vi "heating_visu.vi"(7 "name":string="HT1", 9 "stop":bool, 10 "connect (T)":bool=TRUE, 11 "ZY_In":T4={"Z"={"Z_Source"=enum."local disabled", "Z_SetState"=enum."on", "Z_State"=enum."alarm", "Z_State_T"=0, "ZM_State"=enum."initialization", "ZM_State_T"=0, "ALR  L1"=FALSE, "ALR  L2"=FALSE, "HH_run"=0}, "Y"={"Y_Source"=enum."local disabled", "Y_SetState"=enum."auto", "SP_Set"=0.0, "SP"=0.0, "PV"=0.0, "Y_Set"=0.0, "Y"=0.0, "Y_State"={"code"=0, "visible"=FALSE, "color"=0}, "YB"=FALSE}, "ALR_Status"=[]} {"Y"."Y_Set" format="%.2f"; "Y"."SP" step=0.01 format="%.2f"; "Y"."Y" format="%.2f"; "Y"."PV" step=0.01 format="%.2f"; "Y"."SP_Set" step=0.01 format="%.2f"}) -> (2 "Write Enable":bool, 3 "ZY_out":T1={"Z_HSw"=1, "Z_HSetState"=enum."on", "Y_HSw"=1, "Y_HSetState"=enum."auto", "SP"=0.0, "Y_H"=0.0, "Reset_ALR"=FALSE} {"Y_H" step=1.0; "SP" step=0.01 format="%.2f"}, 5 "This VI":refnum<vi>)   [LabVIEW 2019, in "Heating.lvlib"]
uses:
  Heating.lvlib
  Inputs/Ctl/Parameter State.ctl
  ctl/ZY_state_short.ctl
  ctl/Z.ctl
  ctl/Z_source.ctl
  ctl/Z_State.ctl
  ctl/ZM_State.ctl
  ctl/Y_short.ctl
  ctl/Y_source.ctl
  ctl/Y_state.ctl
  Inputs/Ctl/Parameter State short.ctl
  Alarms/Ctl/ALR_Status_short.ctl
  ctl/ZY_control.ctl
  Logik/fronts.vi
  Trigers/RS.vi
  Trigers/D^.vi
  Timer Delay/Timer.vi
  Counter/Generator simplified.vi
  Global stop.vi
  Change_state.vi
  Timer Delay/Timers.lvlib
  Counter/Counter.lvlib
  Inputs/Inputs.lvlib
  Alarms/Alarms.lvlib
panel:
  in  "on_change":bool
  in  "SP_change":bool
  in  "Y_change":bool
  in  "Z_HSwitch":bool
  out "Z1 ind":u8(ring)
  in  "PV_State":T12
  out "T stage":dbl format="%<%M:%S>t"
  in  "manual control":dbl(slide)=25.0 caption="%" min=0.0 max=100.0 step=1.0 scale=0.0..100.0 scale format="%#.1f"
  out "Z3 ind":u16(ring)
  in  "setpoint":cluster{dbl, dbl}(slide)={350.0, 0.0} caption="oC" scale=0.0..500.0 scale format="%#.1f"
  out "PV":dbl(slide) caption="oC" scale=0.0..500.0 scale format="%#.1f"
  in  "on":bool=TRUE
  in  "ALRL1_reset":bool
  in  "ALRL2_reset":bool
  in  "Y_HSwitch":bool=TRUE
  out "Y ind":u8(ring)
  out "Z5 State":string
  out "Y output":dbl format="%.2f"
  # "PV"
  # "SP"
  # "Y"
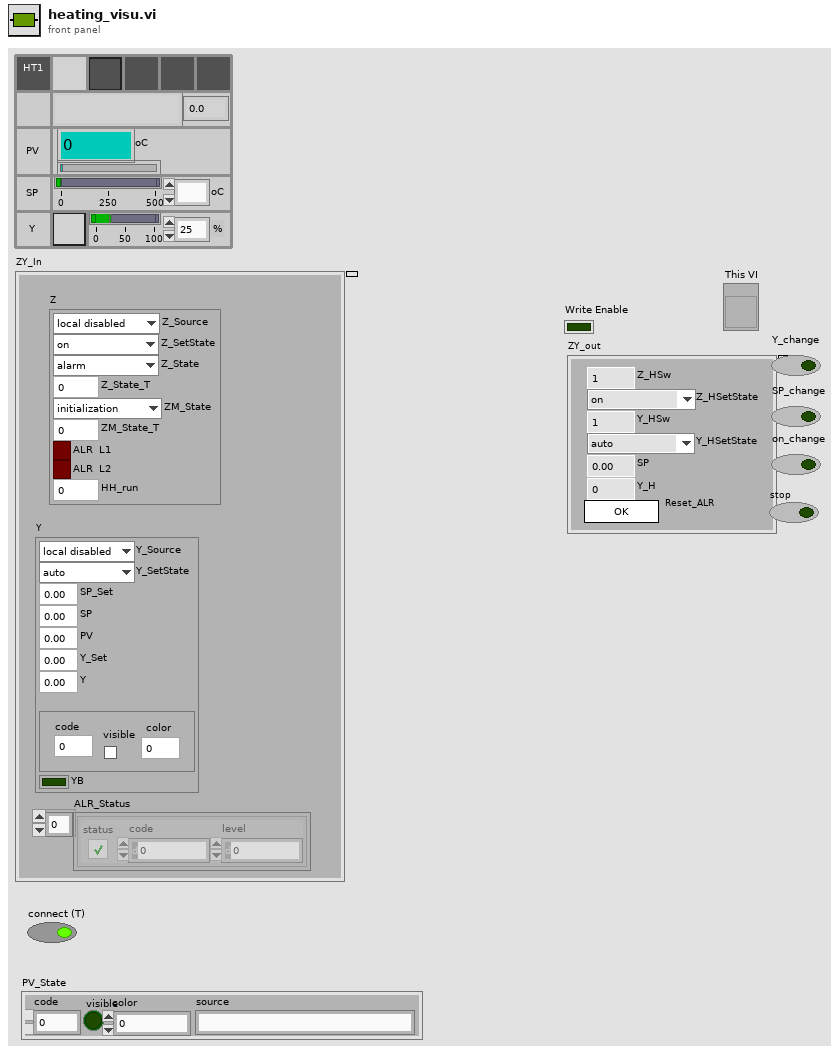
[diagram p1: front panel]
types:
  T1 = typedef "Heating.lvlib/ZY_control.ctl" = cluster{"Z_HSw":u8, "Z_HSetState":T2, "Y_HSw":u8, "Y_HSetState":T3, "SP":dbl, "Y_H":dbl, "Reset_ALR":bool}
  T2 = typedef "Heating.lvlib/Z_State.ctl" = enum8{"initialization", "alarm", "disabled", "not ready", "stop ready", "reserv", "switched off", "reserv2", "switched on", "check", "on min", "decrease out", "on", "increase out", "on max"}
  T3 = typedef "Heating.lvlib/Y_state.ctl" = enum8{"initialize", "alarm", "min", "stop", "hand", "auto", "max"}
  T4 = typedef "Heating.lvlib/ZY_state_short.ctl" = cluster{"Z":T5, "Y":T8, "ALR_Status":T11[]}
  T5 = typedef "Heating.lvlib/Z.ctl" = cluster{"Z_Source":T6, "Z_SetState":T2, "Z_State":T2, "Z_State_T":u32, "ZM_State":T7, "ZM_State_T":u32, "ALR  L1":bool, "ALR  L2":bool, "HH_run":u64}
  T6 = typedef "Heating.lvlib/Z_source.ctl" = enum8{"initialize", "local disabled", "local hand", "hand", "auto", "dist"}
  T7 = typedef "Heating.lvlib/ZM_State.ctl" = enum8{"initialization", "stop", "start_cmd", "contactor_on_cmd", "heating", "on", "stop_cmd", "power_down", "contactor_off_cmd", "cooling", "restart_delay"}
  T8 = typedef "Heating.lvlib/Y_short.ctl" = cluster{"Y_Source":T9, "Y_SetState":T3, "SP_Set":dbl, "SP":dbl, "PV":dbl, "Y_Set":dbl, "Y":dbl, "Y_State":T10, "YB":bool}
  T9 = typedef "Heating.lvlib/Y_source.ctl" = enum8{"initialize", "local disabled", "local hand", "hand", "auto", "dist"}
  T10 = typedef "Inputs.lvlib/Parameter State short.ctl" = cluster{"code":i32, "visible":bool, "color":u32}
  T11 = typedef "Alarms.lvlib/ALR_Status_short.ctl" = cluster{"status":bool, "code":i32, "level":i32}
  T12 = typedef "Inputs.lvlib/Parameter State.ctl" = cluster{"code":i32, "visible":bool, "color":u32, "source":string}
  T13 = enum32{"Invalid Status", "Unconnected", "Active", "Idle", "Error", "Connecting"}
  T14 = enum8{"Enabled", "Disabled", "Disabled and Grayed Out"}
  T15 = typedef "LVDataSocketStatusTypeDef.ctl" = cluster{"Code":enum32{"Invalid Status", "Unconnected", "Active", "Idle", "Error", "Connecting"}, "Text":string}
  T16 = cluster{"Write":bool, "Z1_ind":u8, "Z1_ind_blinking":bool, "Z_HSwitch_out":bool, "Z_HSwitch_visible":bool, "Z_HSwitch_disabled":enum8{"Enabled", "Disabled", "Disabled and Grayed Out"}}
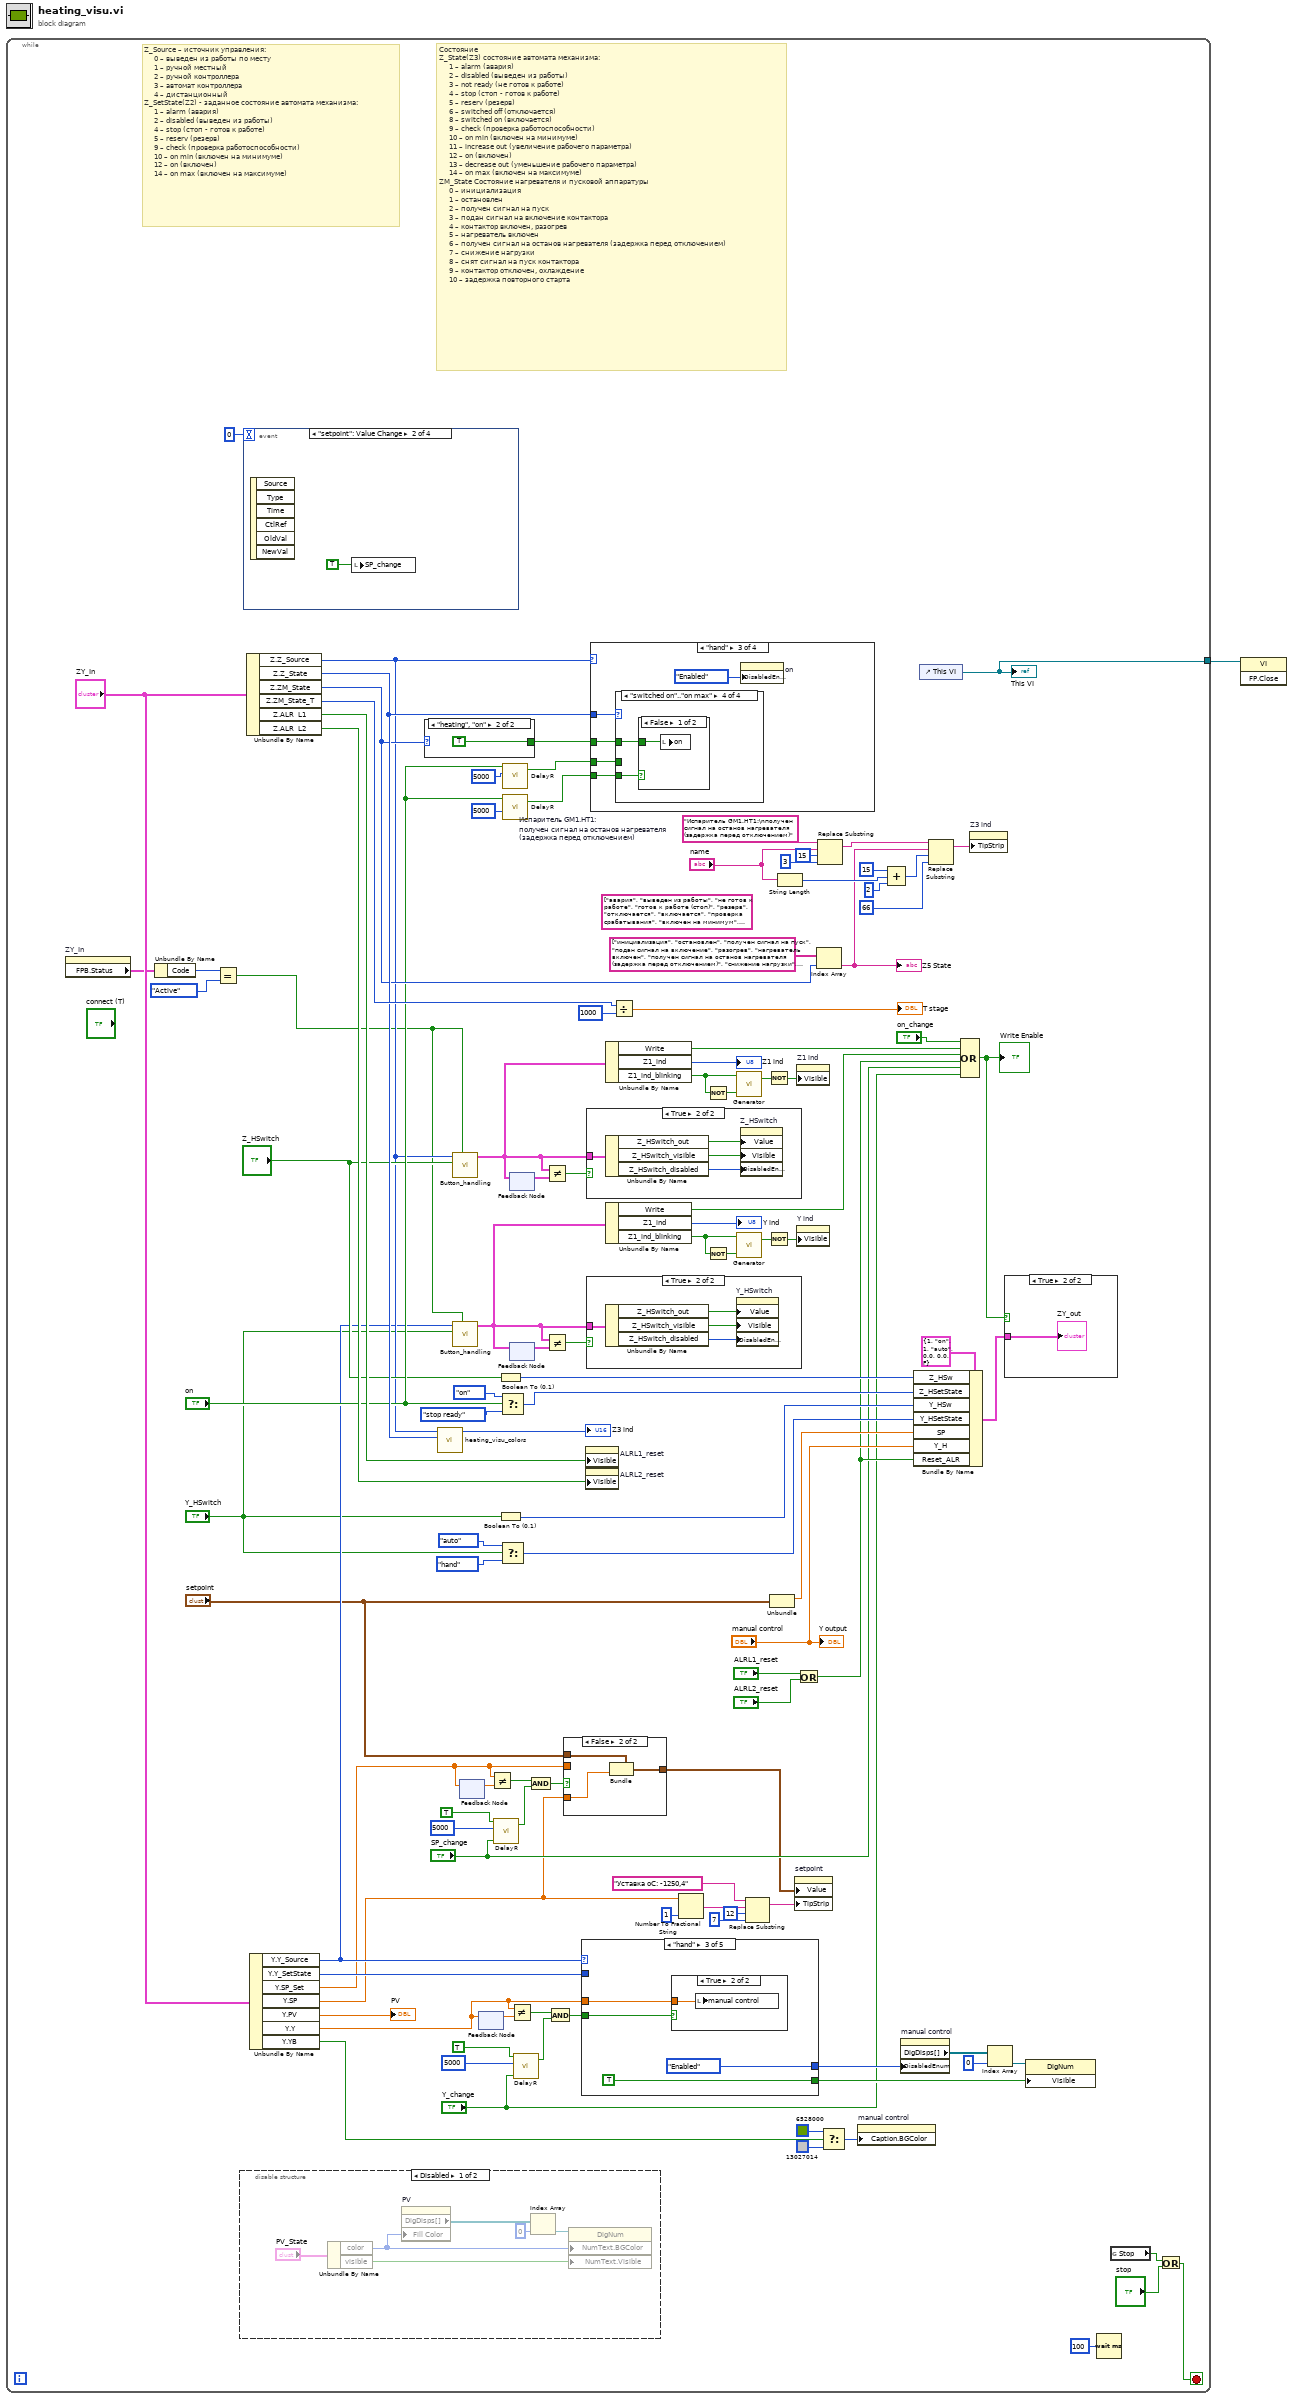
[diagram p0: block diagram]
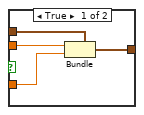
[diagram p3: hidden frame]
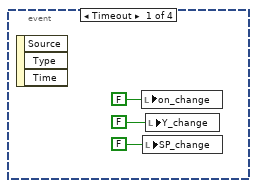
[diagram p4: hidden frame]
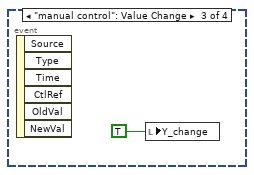
[diagram p5: hidden frame]
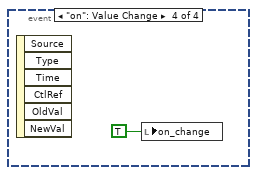
[diagram p6: hidden frame]
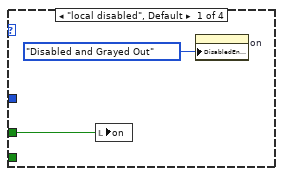
[diagram p8: hidden frame]
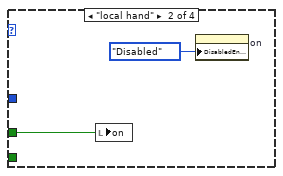
[diagram p9: hidden frame]
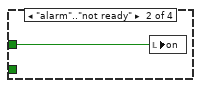
[diagram p11: hidden frame]
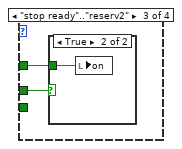
[diagram p12: hidden frame]
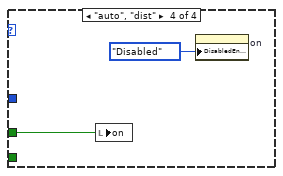
[diagram p15: hidden frame]
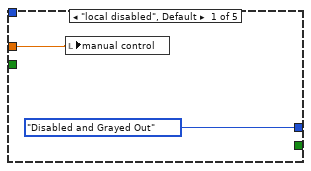
[diagram p19: hidden frame]
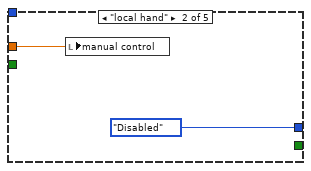
[diagram p20: hidden frame]
diagram:
  n1 = while {
    tunnel: [w2] -> w1
    stop <- w9 stop-if-true
    (unwired) string[] ["авария", "выведен из работы", "не готов к работе", "готов к работе (стоп)", "резерв", "отключается", "включается", "проверка срабатывания", "включен на минимум", "увеличение произв", "включен", "уменьшение произв", "включен на максимум"]
    w106 = "Испаритель GM1.HT1:\nполучен сигнал на останов нагревателя (задержка перед отключением)"  # Испаритель GM1.HT1: получен сигнал на останов нагревателя (задержка перед отключением)
    # "Z_Source – источник управления:\n     0 – выведен из работы по месту\n     1 – ручной местный\n     2 – ручной контроллера\n     3 – автомат контроллера\n     4 – дистанционный\nZ_SetState(Z2) - заданное состояние автомата механизма:\n     1 – alarm (авария)\n     2 – disabled (выведен из работы)\n     4 – stop (стоп - готов к работе)\n     5 – reserv (резерв)\n     9 – check (проверка работоспособности)\n     10 – on min (включен на минимуме)\n     12 – on (включен)\n     14 – on max (включен на максимуме)"
    # "Состояние\nZ_State(Z3) состояние автомата механизма:\n     1 – alarm (авария)\n     2 – disabled (выведен из работы)\n     3 – not ready (не готов к работе)\n     4 – stop (стоп - готов к работе)\n     5 – reserv (резерв)\n     6 – switched off (отключается)\n     8 – switched on (включается)\n     9 – check (проверка работоспособности)\n     10 – on min (включен на минимуме)\n     11 – increase out (увеличение рабочего параметра)\n     12 – on (включен)\n     13 – decrease out (уменьшение рабочего параметра)\n     14 – on max (включен на максимуме)\nZM_State Состояние нагревателя и пусковой аппаратуры\n     0 – инициализация\n     1 – остановлен\n     2 – получен сигнал на пуск\n     3 – подан сигнал на включение контактора\n     4 – контактор включен, разогрев\n     5 – нагреватель включен\n     6 – получен сигнал на останов нагревателя (задержка перед отключением)\n     7 – снижение нагрузки\n     8 – снят сигнал на пуск контактора\n     9 – контактор отключен, охлаждение\n     10 – задержка повторного старта"
    n2 = property on="ZY_In" class="Clust (strict)"() -> ("FPB.Status"=w6:T15)  [unwired: 2 in, 2 out]
    n3 = Unbundle By Name(w6) -> ("Code"=w5:T13)
    n4 = Equal?(x=w5, y=T13."Active" ("Code")) -> (x = y?=w3:bool)
    n5 = disable-structure shown="Disabled" {
      frame Disabled {
        n6 = Unbundle By Name("PV_State") -> ("color"=w156:u32, "visible"=w157:bool)
        n7 = property on="PV" class="Slide (strict)"("Fill Color"=w156) -> ("DigDisps[]"=w160:refnum<vi>[])  [unwired: 2 in, 2 out]
        n8 = Index Array(array=w160, index=0) -> (element=w158:refnum<vi>)
        n9 = property on="Property Node" class="DigNum"(reference=w158, "NumText.BGColor"=w156, "NumText.Visible"=w157) -> ()  [unwired: 1 in, 2 out]
      }
      frame Enabled {
      }
    }
    n10 = event shown="[1] \"setpoint\": Value Change" {
      selector: _ -> [_ _ _ _]
      dyn-events: _ -> [_ _ _ _]
      timeout: 0 -> [_ _ _ _]
      event Timeout {
        n11 = event-data() -> ()  [unwired: 1 in, 3 out]
        n12 = local write "on_change"(FALSE ("manual_reset")) -> ()
        n13 = local write "SP_change"(FALSE ("manual_reset")) -> ()
        n14 = local write "Y_change"(FALSE ("manual_reset")) -> ()
      }
      event "setpoint": Value Change {
        n15 = event-data() -> ()  [unwired: 1 in, 6 out]
        n16 = local write "SP_change"(TRUE ("manual_reset")) -> ()
      }
      event "manual control": Value Change {
        n17 = event-data() -> ()  [unwired: 1 in, 6 out]
        n18 = local write "Y_change"(TRUE ("manual_reset")) -> ()
      }
      event "on": Value Change {
        n19 = event-data() -> ()  [unwired: 1 in, 6 out]
        n20 = local write "on_change"(TRUE ("manual_reset")) -> ()
      }
    }
    n21 = Unbundle By Name("ZY_In") -> ("Z.Z_Source"=w59:T6, "Z.Z_State"=w78:T2, "Z.ZM_State"=w69:T7, "Z.ZM_State_T"=w83:u32, "Z.ALR  L1"=w82:bool, "Z.ALR  L2"=w81:bool)
    n22 = Unbundle By Name("ZY_In") -> ("Y.Y_Source"=w58:T9, "Y.Y_SetState"=w80:T3, "Y.SP_Set"=w19:dbl, "Y.SP"=w16:dbl, "Y.PV"=→"PV":dbl, "Y.Y"=w37:dbl, "Y.YB"=w70:bool)
    n23 = case shown="\"heating\", \"on\"" w69 {
      tunnel: [_ TRUE] -> w88
      frame "initialization", Default {
      }
      frame "heating", "on" {
      }
    }
    n24 = call "heating_visu_colors.vi"("Z_State"=w78, "Z_Source"=w59) -> ("N ring"=→"Z3 ind":u16)  [unwired: 6 in, 3 out]
    n25 = call "Button_handling.vi"("connect"=w3, "Z_HSwitch"="Z_HSwitch", "Z_Source"=w59) -> ("Z_HSwitch_state"=w55:T16)  [unwired: 8 in]
    n26 = call "Button_handling.vi"("connect"=w3, "Z_HSwitch"="Y_HSwitch", "Z_Source"=w58) -> ("Z_HSwitch_state"=w48:T16)  [unwired: 8 in]
    n27 = feedback #1() -> (w28:dbl)  [unwired: 1 in]
    n28 = feedback-in #1(w19) -> ()
    n29 = feedback #2() -> (w39:dbl)  [unwired: 1 in]
    n30 = feedback-in #2(w37) -> ()
    n31 = Not Equal?(x=w19, y=w28) -> (x != y?=w30:bool)
    n32 = call "DelayR.vi"("R"="SP_change", "DelayOn"=u32 5000 ("DelayOff"), "In"=TRUE) -> ("Out"=w31:bool)  [unwired: 1 in, 1 out]
    n33 = Boolean To (0,1)(Boolean="Z_HSwitch") -> (0, 1=w85:i16)
    n34 = Boolean To (0,1)(Boolean="Y_HSwitch") -> (0, 1=w76:i16)
    n35 = Select(t=Z_State."on" ("Z_State"), s="on", f=Z_State."stop ready" ("Z_State")) -> (s? t:f=w89:T2)
    n36 = Select(t=Y_state."auto" ("Y_HSetState"), s="Y_HSwitch", f=Y_state."hand" ("Y_HSetState")) -> (s? t:f=w73:T3)
    n37 = call "DelayR.vi"("DelayOn"=u32 5000 ("DelayOff"), "In"="on") -> ("Out"=w65:bool)  [unwired: 2 in, 1 out]
    n38 = call "DelayR.vi"("DelayOff"=u32 5000, "In"="on") -> ("Out"=w61:bool)  [unwired: 2 in, 1 out]
    n39 = feedback #3() -> (w68:T16)  [unwired: 1 in]
    n40 = feedback-in #3(w55) -> ()
    n41 = feedback #4() -> (w66:T16)  [unwired: 1 in]
    n42 = feedback-in #4(w48) -> ()
    n43 = Not Equal?(x=w37, y=w39) -> (x != y?=w36:bool)
    n44 = call "DelayR.vi"("R"="Y_change", "DelayOn"=u32 5000 ("DelayOff"), "In"=TRUE) -> ("Out"=w35:bool)  [unwired: 1 in, 1 out]
    n45 = And(x=w30, y=w31) -> (x .and. y?=w18:bool)
    n46 = Not Equal?(x=w55, y=w68) -> (x != y?=w56:bool)
    n47 = Not Equal?(x=w48, y=w66) -> (x != y?=w67:bool)
    n48 = And(x=w36, y=w35) -> (x .and. y?=w34:bool)
    n49 = case shown="False" w18 {
      tunnel: w19 -> [w118 _]
      tunnel: [w117 w121] -> w15
      tunnel: "setpoint" -> [w119 w122]
      tunnel: w16 -> [w116 w120]
      frame True {
        n50 = Bundle(cluster=w119, w118, w116) -> (w117:cluster{dbl, dbl})
      }
      frame False {
        n51 = Bundle(cluster=w122, w120) -> (w121:cluster{dbl, dbl})  [unwired: 1 in]
      }
    }
    n52 = case shown="\"hand\"" w58 {
      tunnel: [T14."Disabled and Grayed Out" ("Disabled") T14."Disabled" ("Disabled") T14."Enabled" ("Disabled") T14."Disabled" ("Disabled") T14."Disabled" ("Disabled")] -> w108
      tunnel: [_ _ TRUE _ _] -> w107
      tunnel: w37 -> [w162 w164 w167 w172 w179]
      tunnel: w80 -> [_ _ _ w173 _]
      tunnel: w34 -> [_ _ w166 w171 _]
      frame "local disabled", Default {
        n53 = local write "manual control"(w162) -> ()
      }
      frame "local hand" {
        n54 = local write "manual control"(w164) -> ()
      }
      frame "hand" {
        n55 = case shown="True" w166 {
          tunnel: w167 -> [_ w170]
          frame False {
          }
          frame True {
            n56 = local write "manual control"(w170) -> ()
          }
        }
      }
      frame "auto" {
        n57 = case shown="\"hand\"" w173 {
          tunnel: w172 -> [w176 w178]
          tunnel: w171 -> [w175 _]
          frame "hand" {
            n58 = case shown="True" w175 {
              tunnel: w176 -> [_ w177]
              frame False {
              }
              frame True {
                n59 = local write "manual control"(w177) -> ()
              }
            }
          }
          frame "alarm", Default {
            n60 = local write "manual control"(w178) -> ()
          }
        }
      }
      frame "dist" {
        n61 = local write "manual control"(w179) -> ()
      }
    }
    n62 = property on="ALRL1_reset" class="Bool"("Visible"=w82) -> ()  [unwired: 2 in, 2 out]
    n63 = property on="ALRL2_reset" class="Bool"("Visible"=w81) -> ()  [unwired: 2 in, 2 out]
    n64 = case shown="True" w56 {
      tunnel: w55 -> [_ w151]
      frame False {
      }
      frame True {
        n65 = Unbundle By Name(w151) -> ("Z_HSwitch_out"=w150:bool, "Z_HSwitch_visible"=w149:bool, "Z_HSwitch_disabled"=w148:T14)
        n66 = property on="Z_HSwitch" class="Bool (strict)"("Value"=w150, "Visible"=w149, "DisabledEnum"=w148) -> ()  [unwired: 2 in, 2 out]
      }
    }
    n67 = case shown="True" w67 {
      tunnel: w48 -> [_ w155]
      frame False {
      }
      frame True {
        n68 = Unbundle By Name(w155) -> ("Z_HSwitch_out"=w154:bool, "Z_HSwitch_visible"=w153:bool, "Z_HSwitch_disabled"=w152:T14)
        n69 = property on="Y_HSwitch" class="Bool (strict)"("Value"=w154, "Visible"=w153, "DisabledEnum"=w152) -> ()  [unwired: 2 in, 2 out]
      }
    }
    n70 = case shown="\"hand\"" w59 {
      tunnel: w88 -> [w130 w132 w138 w147]
      tunnel: w78 -> [_ _ w136 _]
      tunnel: w65 -> [_ _ w137 _]
      tunnel: w61 -> [_ _ w134 _]
      frame "local disabled", Default {
        n71 = local write "on"(w130) -> ()
        n72 = property on="on" class="Bool (strict)"("DisabledEnum"=T14."Disabled and Grayed Out" ("Disabled")) -> ()  [unwired: 2 in, 2 out]
      }
      frame "local hand" {
        n73 = local write "on"(w132) -> ()
        n74 = property on="on" class="Bool (strict)"("DisabledEnum"=T14."Disabled" ("Disabled")) -> ()  [unwired: 2 in, 2 out]
      }
      frame "hand" {
        n75 = case shown="\"switched on\"..\"on max\"" w136 {
          tunnel: w138 -> [_ w139 w141 w144]
          tunnel: w137 -> [_ _ w140 _]
          tunnel: w134 -> [_ _ _ w143]
          frame "initialization", Default {
          }
          frame "alarm".."not ready" {
            n76 = local write "on"(w139) -> ()
          }
          frame "stop ready".."reserv2" {
            n77 = case shown="True" w140 {
              tunnel: w141 -> [_ w142]
              frame False {
              }
              frame True {
                n78 = local write "on"(w142) -> ()
              }
            }
          }
          frame "switched on".."on max" {
            n79 = case shown="False" w143 {
              tunnel: w144 -> [w145 _]
              frame False {
                n80 = local write "on"(w145) -> ()
              }
              frame True {
              }
            }
          }
        }
        n81 = property on="on" class="Bool (strict)"("DisabledEnum"=T14."Enabled" ("Disabled")) -> ()  [unwired: 2 in, 2 out]
      }
      frame "auto", "dist" {
        n82 = local write "on"(w147) -> ()
        n83 = property on="on" class="Bool (strict)"("DisabledEnum"=T14."Disabled" ("Disabled")) -> ()  [unwired: 2 in, 2 out]
      }
    }
    n84 = Unbundle By Name(w55) -> ("Write"=w54:bool, "Z1_ind"=→"Z1 ind":u8, "Z1_ind_blinking"=w51:bool)
    n85 = Unbundle By Name(w48) -> ("Write"=w46:bool, "Z1_ind"=→"Y ind":u8, "Z1_ind_blinking"=w50:bool)
    n86 = Divide(x=w83, y=u32 1000) -> (x/y=→"T stage":dbl)
    n87 = Number To Fractional String(number=w16, precision (6)=i16 1) -> (F-format string=w23:string)  [unwired: 2 in]
    n88 = Not(x=w51) -> (.not. x?=w52:bool)
    n89 = Not(x=w50) -> (.not. x?=w49:bool)
    n90 = call "Generator.vi"("R"=w52, "ON (F)"=w51) -> ("Q"=w43:bool)  [unwired: 2 in]
    n91 = call "Generator.vi"("R"=w49, "ON (F)"=w50) -> ("Q"=w45:bool)  [unwired: 2 in]
    n92 = Replace Substring(2:7 ("length (len. of substring)"), 3:12 ("offset (0)"), 4:w23, 5:"Уставка оС: -1250,4") -> (1:w20:string)  [unwired: 1 out]
    n93 = Not(x=w43) -> (.not. x?=w42:bool)
    n94 = Not(x=w45) -> (.not. x?=w44:bool)
    n95 = Unbundle("setpoint") -> (w72:dbl)  [unwired: 1 out]
    n96 = String Length(string="name") -> (length=w100:i32)
    n97 = property on="setpoint" class="Slide (strict)"("Value"=w15, "TipStrip"=w20) -> ()  [unwired: 2 in, 2 out]
    n98 = property on="Z1 ind" class="Ring (strict)"("Visible"=w42) -> ()  [unwired: 2 in, 2 out]
    n99 = property on="Y ind" class="Ring (strict)"("Visible"=w44) -> ()  [unwired: 2 in, 2 out]
    n100 = Or(x="ALRL1_reset", y="ALRL2_reset") -> (x .or. y?=w40:bool)
    n101 = Index Array(array=string[] ["инициализация", "остановлен", "получен сигнал на пуск", "подан сигнал на включение", "разогрев", "нагреватель включен", "получен сигнал на останов нагревателя (задержка перед отключением)", "снижение нагрузки", "снят сигнал на пуск", "охлаждение", "задержка повторного старта"], index=w69) -> (element=w90:string)
    "Z5 State" <- w90
    n102 = Replace Substring(2:3 ("length (len. of substring)"), 3:15 ("offset (0)"), 4:"name", 5:w106) -> (1:w103:string)  [unwired: 1 out]
    n103 = Select(t=u32 6528000, s=w70, f=u32 13027014) -> (s? t:f=w92:u32)
    n104 = property on="manual control" class="Slide (strict)"("Caption.BGColor"=w92) -> ()  [unwired: 2 in, 2 out]
    n105 = Compound Arithmetic op=ADD(15 ("offset (0)"), w100, 2 ("value")) -> (w98:i32)
    n106 = property on="manual control" class="Slide (strict)"("DisabledEnum"=w108) -> ("DigDisps[]"=w113:refnum<vi>[])  [unwired: 2 in, 2 out]
    n107 = Bundle By Name(cluster=T1 {"Z_HSw"=1, "Z_HSetState"=enum."on", "Y_HSw"=1, "Y_HSetState"=enum."auto", "SP"=0.0, "Y_H"=0.0, "Reset_ALR"=FALSE} ("ZY_out"), "Z_HSw"=w85, "Z_HSetState"=w89, "Y_HSw"=w76, "Y_HSetState"=w73, "SP"=w72, "Y_H"="manual control", "Reset_ALR"=w40) -> (w8:T1)
    n108 = control-ref of="This VI"() -> (w2:refnum<vi>)
    "This VI" <- w2
    n109 = Replace Substring(2:66 ("value"), 3:w98, 4:w90, 5:w103) -> (1:w97:string)  [unwired: 1 out]
    n110 = Compound Arithmetic op=OR("on_change", w54, w46, w40, "SP_change", "Y_change") -> (w13:bool)
    "Write Enable" <- w13
    n111 = property on="Z3 ind" class="Ring (strict)"("TipStrip"=w97) -> ()  [unwired: 2 in, 2 out]
    n112 = Index Array(array=w113, index=0) -> (element=w112:refnum<vi>)
    n113 = case shown="True" w13 {
      tunnel: w8 -> [_ w115]
      frame False {
      }
      frame True {
        "ZY_out" <- w115
      }
    }
    n114 = property class="DigNum"(reference=w112, "Visible"=w107) -> ()  [unwired: 1 in, 2 out]
    n115 = Wait (ms)(milliseconds to wait=u32 100) -> ()  [unwired: 1 out]
    n116 = global read "Global stop.vi" "Stop"() -> (w11:bool)
    n117 = Or(x=w11, y="stop") -> (x .or. y?=w9:bool)
    "Y output" <- "manual control"
  }
  n118 = invoke class="VI" method="FP.Close"(reference=w1) -> ()  [unwired: 2 in, 3 out]
